vi "Untitled 4.vi"() -> ()   [LabVIEW 2012]
uses:
  <vilib>/Utility/miscctls.llb/LVRGBAColorTypeDef.ctl
  <vilib>/Utility/miscctls.llb/LV3DPointTypeDef.ctl
  G_DATA.vi
  G_NAV.vi
  <vilib>/picture/3D Picture Control/NI_3D Picture Control.lvlib
panel:
  out "Translation":cluster{"X":sgl, "Y":sgl, "Z":sgl}
  out "appended path":path
  out "3D Picture":refnum<vi>(3d-picture)
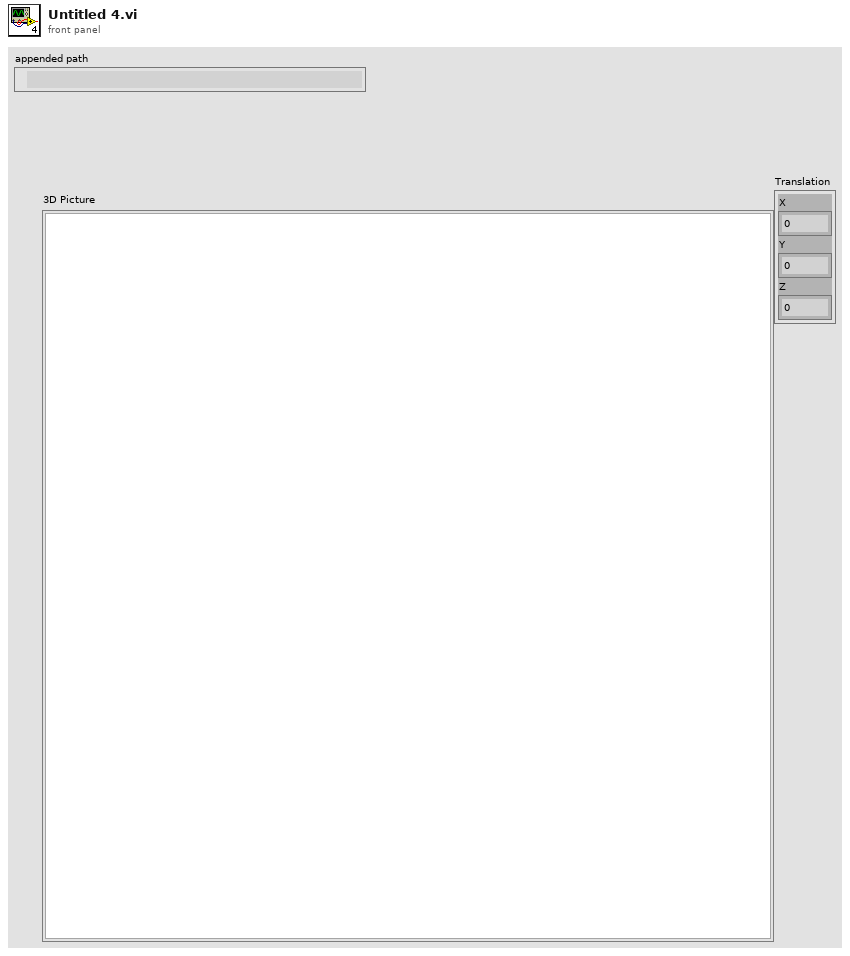
[diagram p1: front panel]
types:
  T1 = cluster{"Red":sgl, "Green":sgl, "Blue":sgl, "Alpha":sgl}
  T2 = enum16{"Overall", "Per Primitive", "Per Vertex", "Binding Off"}
  T3 = typedef "LVRGBAColorTypeDef.ctl" = cluster{"Red":sgl, "Green":sgl, "Blue":sgl, "Alpha":sgl}
  T4 = enum16{"Points", "Lines", "Line Strip", "Line Loop", "Triangles", "Triangle Strip", "Triangle Fan", "Quads", "Quad Strip", "Polygon"}
  T5 = typedef "LV3DPointTypeDef.ctl" = cluster{"X":sgl, "Y":sgl, "Z":sgl}
  T6 = typedef "imagedata.ctl" = cluster{"image type":i32, "image depth":i32, "image":u8[], "mask":u8[], "colors":u32[], "Rectangle":cluster{"left":i16, "top":i16, "right":i16, "bottom":i16}}
  T7 = cluster{"left":i16, "top":i16, "right":i16, "bottom":i16}
  T8 = cluster{"left":sgl, "top":sgl, "right":sgl, "bottom":sgl}
  T9 = enum16{"None", "Spherical", "Flying", "Oriented"}
  T10 = cluster{"GPSTime":dbl, "attitude[2]":dbl, "lcc[0]":dbl, "lcc[1]":dbl, "heading_GPS":dbl}
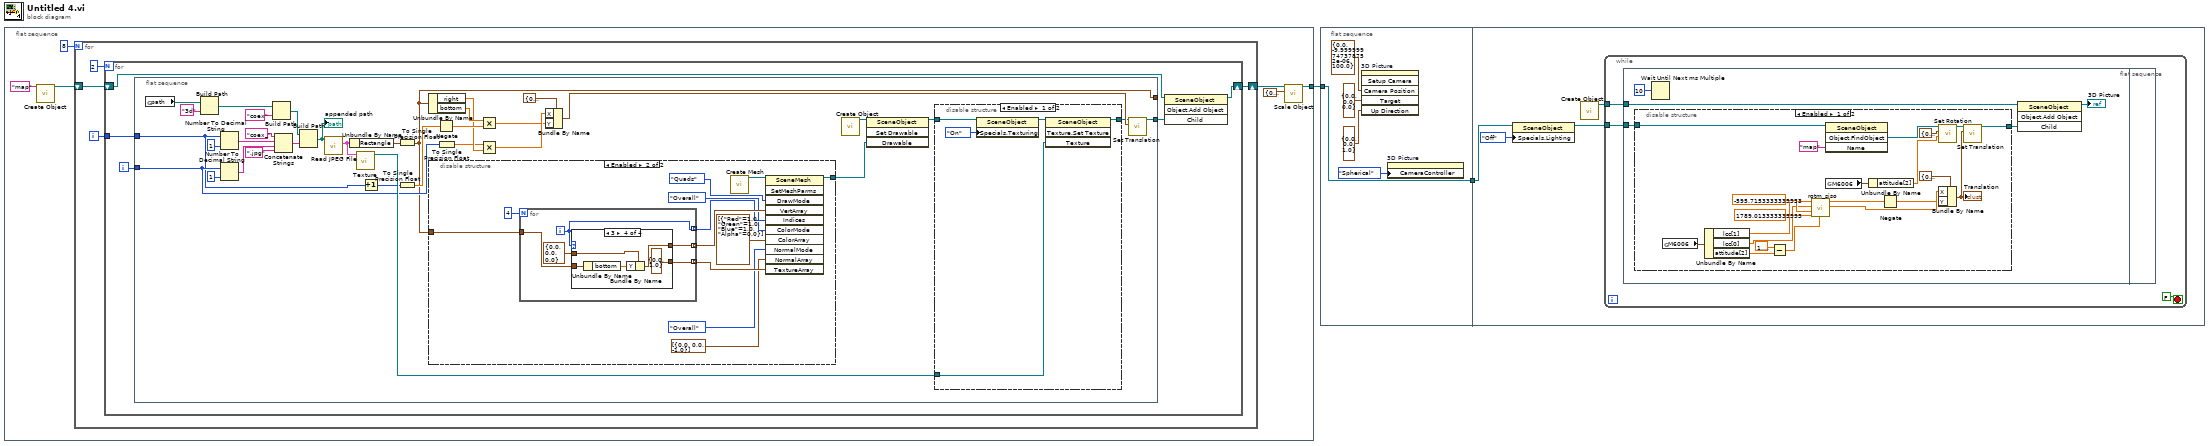
[diagram p0: block diagram]
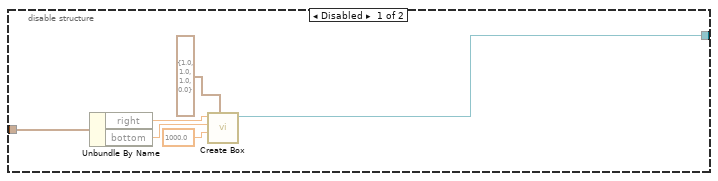
[diagram p3: hidden frame]
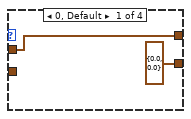
[diagram p4: hidden frame]
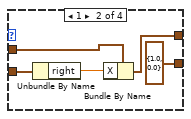
[diagram p5: hidden frame]
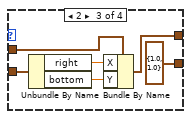
[diagram p6: hidden frame]
diagram:
  n1 = flat-sequence {
    tunnel: [w4] -> w1
    frame #0 {
      n2 = call <vilib>:"Create Object.vi"("Name"="map") -> ("Scene:New Object"=w5:refnum<vi>)  [unwired: 1 in, 9 out]
      n3 = for {
        N: 8 -> [_]
        shift-right: [w10] -> w3
        shift-left: w5 -> [w12]
        i -> [w9]
        n4 = for {
          N: 2 -> [_]
          shift-right: [w15] -> w10
          shift-left: w12 -> [w17]
          tunnel: w9 -> [w13]
          i -> [w14]
          n5 = flat-sequence {
            tunnel: [w32] -> w16
            tunnel: w14 -> [w31]
            tunnel: w13 -> [w20]
            tunnel: [w23] -> _
            frame #0 {
              n6 = global read "G_DATA.vi" "path"() -> (w47:path)
              n7 = Build Path(base path=w47, name or relative path="3d") -> (appended path=w45:path)
              n8 = Number To Decimal String(number=w20, width (-)=i16 1) -> (decimal integer string=w24:string)
              n9 = Number To Decimal String(number=w31, width (-)=i16 1) -> (decimal integer string=w38:string)
              n10 = Build Path(base path=w45, name or relative path="coex") -> (appended path=w43:path)
              n11 = Concatenate Strings("coex_" ("string"), w24, w38, ".jpg" ("name or relative path")) -> (w36:string)
              n12 = Build Path(base path=w43, name or relative path=w36) -> (appended path=w42:path)
              "appended path" <- w42
              n13 = call <vilib>:"Read JPEG File.vi"("path to JPEG file"=w42) -> ("image data"=w41:T6)  [unwired: 8 in, 2 out]
              n14 = Unbundle By Name(w41) -> ("Rectangle"=w40:T7)
              n15 = call <vilib>:"Texture.vi"("Image"=w41) -> ("New Texture Refnum"=w51:refnum<vi>)  [unwired: 1 in, 9 out]
              n16 = Increment(x=w20) -> (x+1=w19:i32)
              n17 = To Single Precision Float(number=w40) -> (single precision float=w23:T8)
              n18 = To Single Precision Float(number=w19) -> (single precision float=w29:sgl)
              n19 = Unbundle By Name(w23) -> ("right"=w22:sgl, "bottom"=w28:sgl)
              n20 = disable-structure shown="Enabled" {
                disable-tunnel: [w62 w74] -> w48
                disable-tunnel: w23 -> [w58 w69]
                frame Disabled {
                  n21 = Unbundle By Name(w58) -> ("right"=w60:sgl, "bottom"=w59:sgl)
                  n22 = call <vilib>:"Create Box.vi"("Color"=T1 {"Red"=1.0, "Green"=1.0, "Blue"=1.0, "Alpha"=0.0}, "Length Z"=sgl 1000.0, "Length Y"=w59, "Length X"=w60) -> ("New Box Refnum"=w62:refnum<vi>)  [unwired: 6 in, 1 out]
                }
                frame Enabled {
                  n23 = for {
                    N: 4 -> [_]
                    tunnel: [w79] -> w71 mode=indexing
                    tunnel: [w78] -> w70 mode=indexing
                    tunnel: w69 -> [w77]
                    tunnel: [w76] -> w66 mode=indexing
                    i -> [w78]
                    n24 = case shown="3" w78 {
                      tunnel: T5 {"X"=0.0, "Y"=0.0, "Z"=0.0} ("3D Point") -> [w82 w87 w93 w98]
                      tunnel: [w82 w86 w92 w97] -> w79
                      tunnel: w77 -> [_ w85 w91 w96]
                      tunnel: [cluster{"S":sgl, "T":sgl} {"S"=0.0, "T"=0.0} cluster{"S":dbl, "T":sgl} {"S"=1.0, "T"=0.0} cluster{"S":dbl, "T":dbl} {"S"=1.0, "T"=1.0} cluster{"S":dbl, "T":dbl} {"S"=0.0, "T"=1.0}] -> w76
                      frame 0, Default {
                      }
                      frame 1 {
                        n25 = Unbundle By Name(w85) -> ("right"=w84:sgl)
                        n26 = Bundle By Name(cluster=w87, "X"=w84) -> (w86:T5)
                      }
                      frame 2 {
                        n27 = Unbundle By Name(w91) -> ("right"=w90:sgl, "bottom"=w89:sgl)
                        n28 = Bundle By Name(cluster=w93, "X"=w90, "Y"=w89) -> (w92:T5)
                      }
                      frame 3 {
                        n29 = Unbundle By Name(w96) -> ("bottom"=w95:sgl)
                        n30 = Bundle By Name(cluster=w98, "Y"=w95) -> (w97:T5)
                      }
                    }
                  }
                  n31 = call <vilib>:"Create Mesh.vi"() -> ("New Mesh Refnum"=w75:refnum<vi>)  [unwired: 10 in, 1 out]
                  n32 = invoke class="SceneMesh" method="SetMeshParms"(reference=w75, "DrawMode"=T4."Quads" ("Draw Mode"), "VertArray"=w71, "Indices"=w70, "ColorMode"=T2."Overall" ("Color Binding Mode"), "ColorArray"=T3[] [{"Red"=1.0, "Green"=1.0, "Blue"=1.0, "Alpha"=0.0}] ("Color Array"), "NormalMode"=T2."Overall" ("Normal Binding Mode"), "NormalArray"=cluster{"X":sgl, "Y":sgl, "Z":sgl}[] [{"X"=0.0, "Y"=0.0, "Z"=-1.0}], "TextureArray"=w66) -> (reference out=w74:refnum<vi>)  [unwired: 2 in, 10 out]
                }
              }
              n33 = Negate(x=w29) -> (-x=w27:sgl)
              n34 = To Single Precision Float(number=w31) -> (single precision float=w21:sgl)
              n35 = Multiply(x=w28, y=w27) -> (x*y=w26:sgl)
              n36 = Multiply(x=w21, y=w22) -> (x*y=w34:sgl)
              n37 = Bundle By Name(cluster=cluster{"X":sgl, "Y":sgl, "Z":sgl} {"X"=0.0, "Y"=0.0, "Z"=0.0} ("Translation"), "X"=w34, "Y"=w26) -> (w33:cluster{"X":sgl, "Y":sgl, "Z":sgl})
              n38 = call <vilib>:"Create Object.vi"() -> ("Scene:New Object"=w49:refnum<vi>)  [unwired: 2 in, 9 out]
              n39 = invoke class="SceneObject" method="Set Drawable"(reference=w49, "Drawable"=w48) -> (reference out=w50:refnum<vi>)  [unwired: 2 in, 3 out]
              n40 = disable-structure shown="Enabled" {
                disable-tunnel: w51 -> [w56 _]
                disable-tunnel: w50 -> [w54 w57]
                disable-tunnel: [w52 w57] -> w18
                frame Enabled {
                  n41 = property class="SceneObject"(reference=w54, "Specials.Texturing"=enum16{"Inherit Value", "Off", "On"}."On" ("Specials:Texturing")) -> (reference out=w53:refnum<vi>)  [unwired: 1 in, 1 out]
                  n42 = invoke class="SceneObject" method="Texture.Set Texture"(reference=w53, "Texture"=w56) -> (reference out=w52:refnum<vi>)  [unwired: 2 in, 3 out]
                }
                frame Disabled {
                }
              }
              n43 = call <vilib>:"Set Translation.vi"("Translation"=w33, "Scene Object"=w18) -> ("Translated Object"=w32:refnum<vi>)  [unwired: 8 in, 1 out]
            }
          }
          n44 = invoke class="SceneObject" method="Object.Add Object"(reference=w17, "Child"=w16) -> (reference out=w15:refnum<vi>)  [unwired: 2 in, 3 out]
        }
      }
      n45 = call <vilib>:"Scale Object.vi"("Scale"=cluster{"X":sgl, "Y":sgl, "Z":sgl} {"X"=0.16666667, "Y"=0.16666667, "Z"=0.16666667}, "Scene.Object In"=w3) -> ("Scene.Object Out"=w4:refnum<vi>)  [unwired: 8 in, 1 out]
    }
  }
  n46 = flat-sequence {
    tunnel: w1 -> [w103]
    tunnel: [w103] -> w2
    tunnel: w2 -> [w106]
    frame #0 {
      n47 = invoke on="3D Picture" class="SceneGraphDisp (strict)" method="Setup Camera"("Camera Position"=cluster{"X":sgl, "Y":sgl, "Z":sgl} {"X"=0.0, "Y"=-1e-05, "Z"=100.0}, "Target"=cluster{"X":sgl, "Y":sgl, "Z":sgl} {"X"=0.0, "Y"=0.0, "Z"=0.0}, "Up Direction"=cluster{"X":sgl, "Y":sgl, "Z":sgl} {"X"=0.0, "Y"=0.0, "Z"=1.0}) -> ()  [unwired: 3 in, 6 out]
      n48 = property on="3D Picture" class="SceneGraphDisp (strict)"("CameraController"=T9."Spherical" ("Camera Controller:Type")) -> ()  [unwired: 2 in, 2 out]
    }
    frame #1 {
      n49 = property class="SceneObject"(reference=w106, "Specials.Lighting"=enum16{"Inherit Value", "Off", "On"}."Off" ("Specials:Lighting")) -> (reference out=w105:refnum<vi>)  [unwired: 1 in, 1 out]
      n50 = call <vilib>:"Create Object.vi"() -> ("Scene:New Object"=w104:refnum<vi>)  [unwired: 2 in, 9 out]
      n51 = while {
        tunnel: w105 -> [w110]
        tunnel: w104 -> [w109]
        stop <- FALSE stop-if-true
        n52 = flat-sequence {
          tunnel: w110 -> [w114]
          tunnel: w109 -> [w113]
          frame #0 {
            n53 = disable-structure shown="Enabled" {
              disable-tunnel: w114 -> [w133 w137]
              disable-tunnel: [w134 w137] -> w112
              frame Enabled {
                n54 = global read "G_NAV.vi" "M6006"() -> (w136:T10)
                n55 = Unbundle By Name(w136) -> ("lcc[1]"=w123:dbl, "lcc[0]"=w122:dbl, "attitude[2]"=w126:dbl)
                n56 = Subtract(x=1.5707963267948966, y=w126) -> (x-y=w127:dbl)
                n57 = call "rotm_siso.vi"("angle[rad]"=w127, "y0"=1789.013333333333, "x0"=-595.7153333333333, "y"=w122, "x"=w123) -> ("y'"=w121:dbl, "x'"=w120:dbl)  [unwired: 5 in]
                n58 = invoke class="SceneObject" method="Object.FindObject"(reference=w133, "Name"="map") -> ("FindObject"=w129:refnum<vi>)  [unwired: 2 in, 3 out]
                n59 = global read "G_NAV.vi" "M6006"() -> (w117:T10)
                n60 = Unbundle By Name(w117) -> ("attitude[2]"=w116:dbl)
                n61 = Negate(x=w120) -> (-x=w119:dbl)
                n62 = call <vilib>:"Set Rotation.vi"("Angle"=w116, "Axis"=cluster{"X":sgl, "Y":sgl, "Z":sgl} {"X"=0.0, "Y"=0.0, "Z"=1.0}, "Scene Object"=w129) -> ("Rotated Scene Object"=w131:refnum<vi>)  [unwired: 7 in, 1 out]
                n63 = Bundle By Name(cluster=cluster{"X":sgl, "Y":sgl, "Z":sgl} {"X"=0.0, "Y"=0.0, "Z"=0.0} ("Translation"), "X"=w121, "Y"=w119) -> (w130:cluster{"X":sgl, "Y":sgl, "Z":sgl})
                "Translation" <- w130
                n64 = call <vilib>:"Set Translation.vi"("Translation"=w130, "Scene Object"=w131) -> ("Translated Object"=w134:refnum<vi>)  [unwired: 8 in, 1 out]
              }
              frame Disabled {
              }
            }
            n65 = Wait Until Next ms Multiple(millisecond multiple=u32 10) -> ()  [unwired: 1 out]
            n66 = invoke class="SceneObject" method="Object.Add Object"(reference=w113, "Child"=w112) -> (reference out=→"3D Picture":refnum<vi>)  [unwired: 2 in, 3 out]
          }
          frame #1 {
          }
        }
      }
    }
  }
